vi "SPI Write Read.vi"   [LabVIEW 2011, in "LVH-LINX.lvlib"]
uses:
  LVH-LINX.lvlib
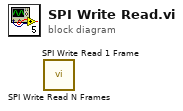
[diagram p0: block diagram]
diagram:
  n1 = call "SPI Write Read N Frames.vi"() -> ()  [unwired: 9 in, 3 out]
  n2 = call "SPI Write Read 1 Frame.vi"() -> ()  [unwired: 9 in, 3 out]
